vi "Image_Set ColorSpace.vi"(0 "Image_3d":u8[][][](array[numeric]), 5 "error in (no error)":errorcluster, 7 "ColorSpace":T1) -> (12 "tick(ms)":u32, 14 "Image_3d_ColorSpace":u8[][][](array[numeric]), 19 "error out":errorcluster)   [LabVIEW 2016]
uses:
  Typedefs/typedef_enum_ColorSpace.ctl
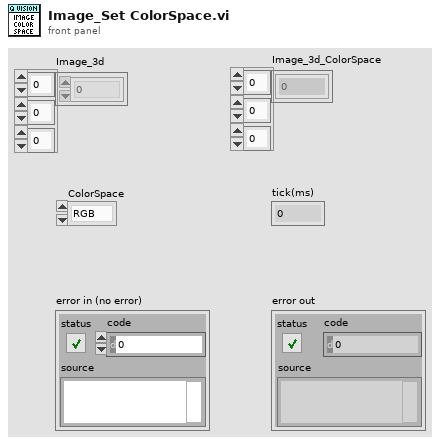
[diagram p1: front panel]
types:
  T1 = typedef "typedef_enum_ColorSpace.ctl" = enum16{"RGB", "HSL"}
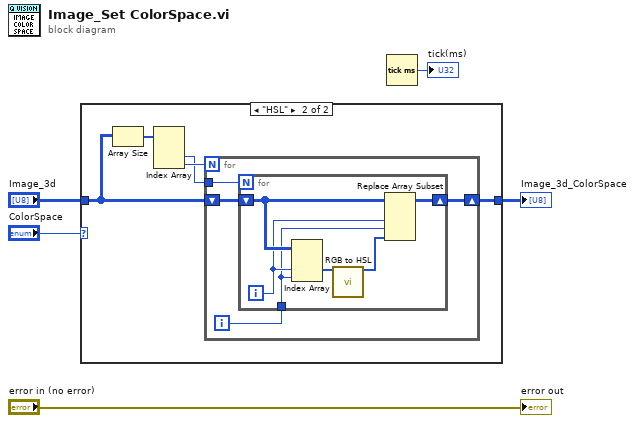
[diagram p0: block diagram]
diagram:
  n1 = case shown="\"HSL\"" "ColorSpace" {
    tunnel: [w6 w11] -> w4
    tunnel: "Image_3d" -> [w6 w10]
    frame "RGB", Default {
    }
    frame "HSL" {
      n2 = Array Size(array=w10) -> (size(s)=w9:i32[])
      n3 = Index Array(array=w9) -> (element #2=w7:i32, element #3=w8:i32)  [unwired: 3 in, 1 out]
      n4 = for {
        N: w8 -> [_]
        shift-right: [w13] -> w11
        shift-left: w10 -> [w15]
        tunnel: w7 -> [w12]
        i -> [w14]
        n5 = for {
          N: w12 -> [_]
          tunnel: w14 -> [w18]
          shift-right: [w16] -> w13
          shift-left: w15 -> [w20]
          i -> [w19]
          n6 = Index Array(array=w20, index (dim 1)=w19, index (dim 2)=w18) -> (element=w21:u8[])  [unwired: 1 in]
          n7 = call "RGB to HSL.vi"("RGB"=w21) -> ("HSL"=w17:u8[])  [unwired: 14 in]
          n8 = Replace Array Subset(array=w20, new element=w17, index (dim 1)=w19, index (dim 2)=w18) -> (w16:u8[][][])  [unwired: 1 in]
        }
      }
    }
  }
  "Image_3d_ColorSpace" <- w4
  n9 = Tick Count (ms)() -> (millisecond timer value=→"tick(ms)":u32)
  "error out" <- "error in (no error)"
